vi "Cubo_Color.vi"() -> ()   [LabVIEW 2016]
panel:
  out "new picture 6":picture
  out "new picture 5":picture
  out "new picture 4":picture
  out "new picture 3":picture
  out "new picture 2":picture
  out "new picture":picture
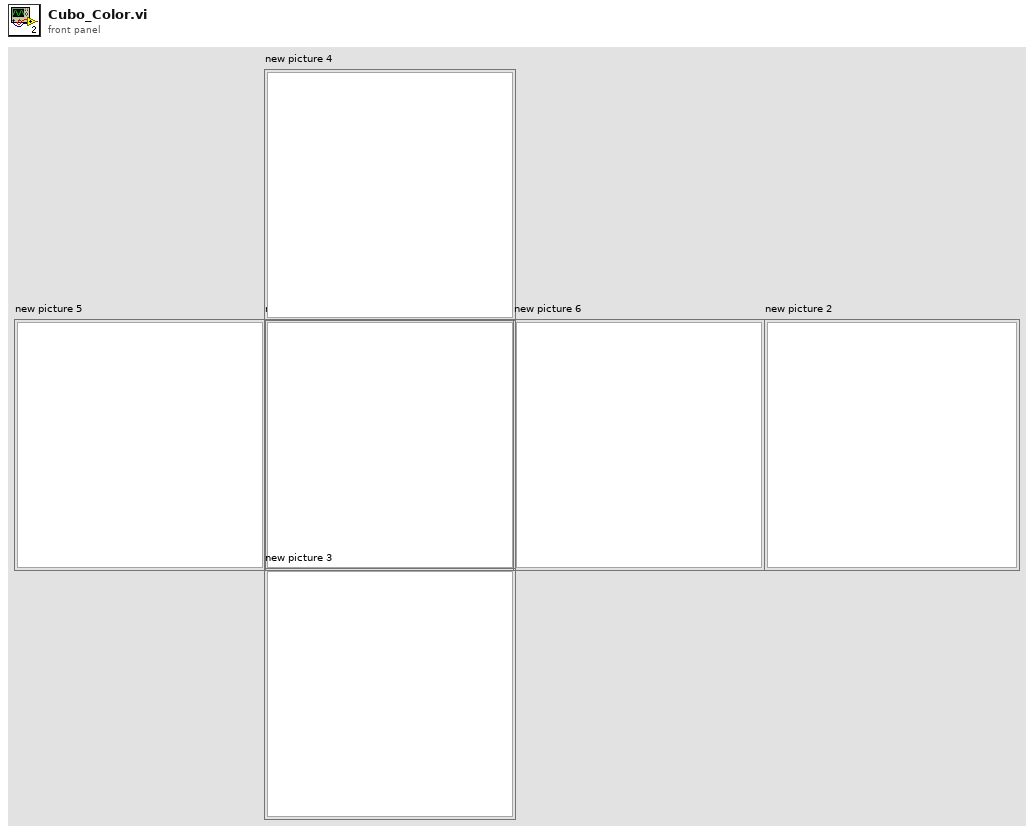
[diagram p1: front panel]
types:
  T1 = typedef "imagedata.ctl" = cluster{"image type":i32, "image depth":i32, "image":u8[], "mask":u8[], "colors":u32[], "Rectangle":cluster{"left":i16, "top":i16, "right":i16, "bottom":i16}}
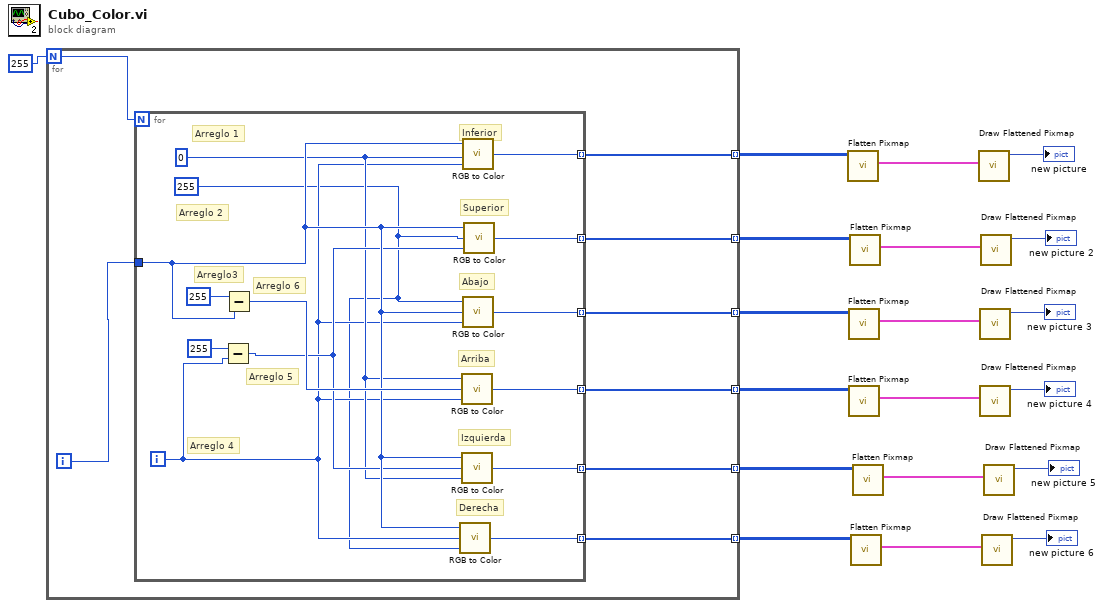
[diagram p0: block diagram]
diagram:
  n1 = for {
    N: u8 255 -> [w27]
    tunnel: [w25] -> w6 mode=indexing
    tunnel: [w24] -> w5 mode=indexing
    tunnel: [w23] -> w4 mode=indexing
    tunnel: [w22] -> w3 mode=indexing
    tunnel: [w21] -> w2 mode=indexing
    tunnel: [w20] -> w1 mode=indexing
    i -> [w26]
    n2 = for {
      N: w27 -> [_]
      tunnel: w26 -> [w38]
      tunnel: [w33] -> w25 mode=indexing
      tunnel: [w32] -> w24 mode=indexing
      tunnel: [w31] -> w23 mode=indexing
      tunnel: [w30] -> w22 mode=indexing
      tunnel: [w29] -> w21 mode=indexing
      tunnel: [w28] -> w20 mode=indexing
      i -> [w35]
      w34 = u8 255
      w36 = u8 0 ("x")
      # "Arreglo3"
      # "Arreglo 4"
      # "Derecha"
      # "Izquierda"
      # "Arriba"
      # "Abajo"
      # "Superior"
      # "Inferior"
      # "Arreglo 5"
      # "Arreglo 6"
      # "Arreglo 1"
      # "Arreglo 2"
      n3 = Subtract(x=u8 255, y=w35) -> (x-y=w37:i32)
      n4 = Subtract(x=u8 255, y=w38) -> (x-y=w39:i32)
      n5 = call <vilib>:"RGB to Color.vi"("B"=w34, "G"=w35, "R"=w38) -> ("Color"=w28:u32)
      n6 = call <vilib>:"RGB to Color.vi"("B"=w35, "G"=w39, "R"=w36) -> ("Color"=w30:u32)
      n7 = call <vilib>:"RGB to Color.vi"("B"=w36, "G"=w37, "R"=w38) -> ("Color"=w29:u32)
      n8 = call <vilib>:"RGB to Color.vi"("B"=w35, "G"=w36, "R"=w38) -> ("Color"=w33:u32)
      n9 = call <vilib>:"RGB to Color.vi"("B"=w35, "G"=w38, "R"=w34) -> ("Color"=w31:u32)
      n10 = call <vilib>:"RGB to Color.vi"("B"=w37, "G"=w34, "R"=w38) -> ("Color"=w32:u32)
    }
  }
  n11 = call <vilib>:"Flatten Pixmap.vi"("24-bit pixmap"=w6) -> ("image data"=w18:T1)  [unwired: 10 in]
  n12 = call <vilib>:"Flatten Pixmap.vi"("24-bit pixmap"=w4) -> ("image data"=w13:T1)  [unwired: 10 in]
  n13 = call <vilib>:"Flatten Pixmap.vi"("24-bit pixmap"=w3) -> ("image data"=w12:T1)  [unwired: 10 in]
  n14 = call <vilib>:"Flatten Pixmap.vi"("24-bit pixmap"=w5) -> ("image data"=w16:T1)  [unwired: 10 in]
  n15 = call <vilib>:"Flatten Pixmap.vi"("24-bit pixmap"=w1) -> ("image data"=w8:T1)  [unwired: 10 in]
  n16 = call <vilib>:"Flatten Pixmap.vi"("24-bit pixmap"=w2) -> ("image data"=w9:T1)  [unwired: 10 in]
  n17 = call <vilib>:"Draw Flattened Pixmap.vi"("image data"=w18) -> ("new picture"=→"new picture":picture)  [unwired: 8 in]
  n18 = call <vilib>:"Draw Flattened Pixmap.vi"("image data"=w13) -> ("new picture"=→"new picture 3":picture)  [unwired: 8 in]
  n19 = call <vilib>:"Draw Flattened Pixmap.vi"("image data"=w12) -> ("new picture"=→"new picture 4":picture)  [unwired: 8 in]
  n20 = call <vilib>:"Draw Flattened Pixmap.vi"("image data"=w16) -> ("new picture"=→"new picture 2":picture)  [unwired: 8 in]
  n21 = call <vilib>:"Draw Flattened Pixmap.vi"("image data"=w8) -> ("new picture"=→"new picture 6":picture)  [unwired: 8 in]
  n22 = call <vilib>:"Draw Flattened Pixmap.vi"("image data"=w9) -> ("new picture"=→"new picture 5":picture)  [unwired: 8 in]
